vi "Visible and Boolean Text Properties.vi"(0 "Control References":refnum<vi>[](array[refnum]), 2 "Option":enum16{"Visible", "Boolean Text"}(ring)=enum."Boolean Text", 5 "error in (no error)":errorcluster, 6 "Boolean Text Array":string[](array[string]), 8 "Controls Visible Property Values":bool[](array[boolean])) -> (19 "error out":errorcluster)   [LabVIEW 2015]
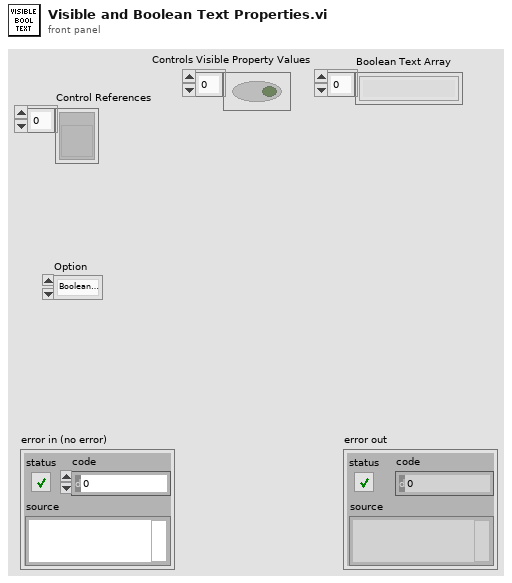
[diagram p1: front panel]
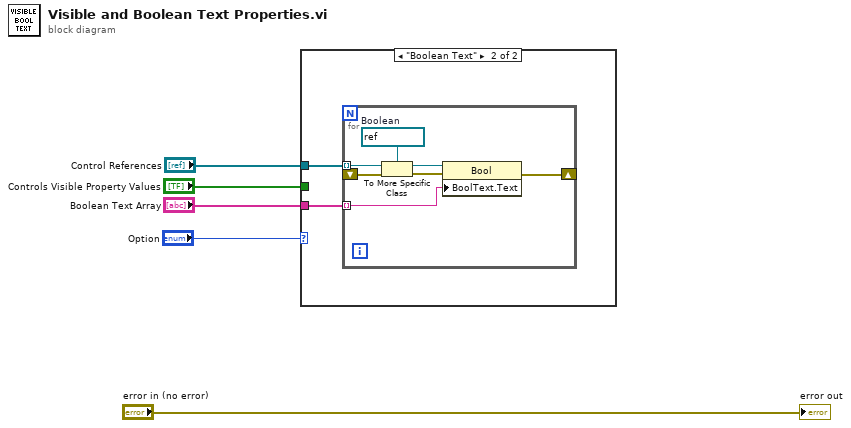
[diagram p0: block diagram]
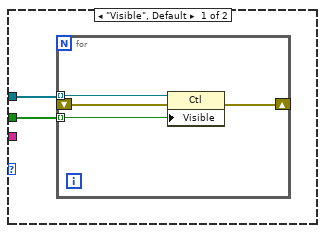
[diagram p2: hidden frame]
diagram:
  n1 = case shown="\"Boolean Text\"" "Option" {
    tunnel: "Control References" -> [w7 w13]
    tunnel: "Controls Visible Property Values" -> [w6 _]
    tunnel: "Boolean Text Array" -> [_ w12]
    frame "Visible", Default {
      n2 = for {
        tunnel: w7 -> [w11] mode=indexing
        shift-right: [w9] -> _
        shift-left: _ -> [w10]
        tunnel: w6 -> [w8] mode=indexing
        n3 = property class="Ctl"(reference=w11, error in=w10, "Visible"=w8) -> (error out=w9:errorcluster)  [unwired: 1 out]
      }
    }
    frame "Boolean Text" {
      n4 = for {
        tunnel: w13 -> [w20] mode=indexing
        shift-right: [w16] -> _
        shift-left: _ -> [w15]
        tunnel: w12 -> [w14] mode=indexing
        w18 = refnum<vi> refnum  # Boolean
        n5 = To More Specific Class(target class=w18, reference=w20, error in=w15) -> (specific class reference=w19:refnum<vi>, error out=w17:errorcluster)
        n6 = property class="Bool"(reference=w19, error in=w17, "BoolText.Text"=w14) -> (error out=w16:errorcluster)  [unwired: 1 out]
      }
    }
  }
  "error out" <- "error in (no error)"
